vi "zero_voltage!.vi"(0 "Voltages":dbl[](array[numeric]) format="%_6f") -> ()   [LabVIEW 2010]
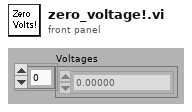
[diagram p1: front panel]
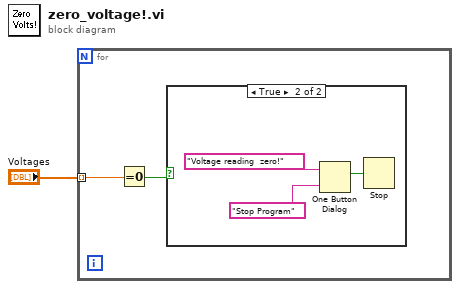
[diagram p0: block diagram]
diagram:
  n1 = for {
    tunnel: "Voltages" -> [w2] mode=indexing
    n2 = Equal To 0?(x=w2) -> (x = 0?=w3:bool)
    n3 = case shown="True" w3 {
      frame False {
      }
      frame True {
        n4 = One Button Dialog(message="Voltage reading  zero!", button name ("OK")="Stop Program") -> (true=w4:bool)
        n5 = Stop(stop? (T)=w4) -> ()
      }
    }
  }
